vi "Do.vi"(8 "error in (no error)":errorcluster, 10 "Actor in":refnum<class "Actor.lvclass">, 11 "Stop Msg":refnum<class "Proxy Stop Msg.lvclass">) -> (0 "error out":errorcluster, 2 "Actor out":refnum<class "Actor.lvclass">)   [LabVIEW 2014, in "Proxy.lvlib" / "Proxy Stop Msg.lvclass"]
uses:
  Proxy Stop Msg.lvclass
  <vilib>/ActorFramework/Actor/Actor.lvclass
  Proxy Stop Msg.lvclass/Proxy Stop Msg.ctl
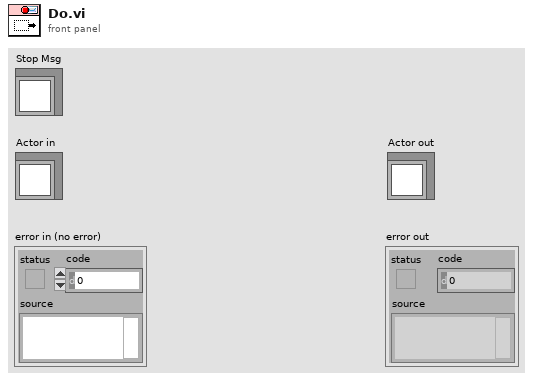
[diagram p1: front panel]
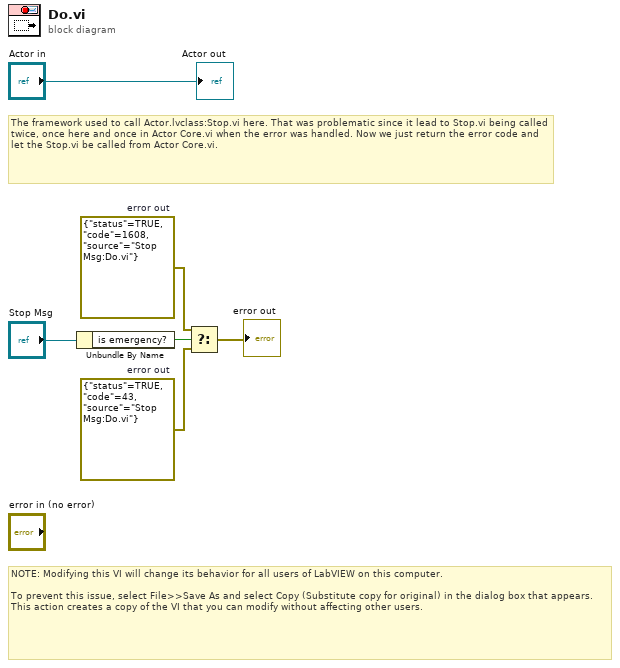
[diagram p0: block diagram]
diagram:
  w1 = errorcluster {"status"=TRUE, "code"=43, "source"="Stop Msg:Do.vi"}  # error out
  w2 = errorcluster {"status"=TRUE, "code"=1608, "source"="Stop Msg:Do.vi"}  # error out
  # "NOTE: Modifying this VI will change its behavior for all users of LabVIEW on this computer.\n\nTo prevent this issue, select File>>Save As and select Copy (Substitute copy for original) in the dialog box that appears. This action creates a copy of the VI that you can modify without affecting other users."
  # "The framework used to call Actor.lvclass:Stop.vi here. That was problematic since it lead to Stop.vi being called twice, once here and once in Actor Core.vi when the error was handled. Now we just return the error code and let the Stop.vi be called from Actor Core.vi."
  n1 = Unbundle By Name("Stop Msg") -> ("is emergency?"=w4:bool)
  n2 = Select(t=w2, s=w4, f=w1) -> (s? t:f=→"error out":errorcluster)
  "Actor out" <- "Actor in"
